vi "Periodic Tasks.vi"(8 "error in":errorcluster) -> ()   [LabVIEW 2013]
doc: "This VI runs in parallel to other tasks. It can contain as many user-defined periodic loops as you need. These can carry out PID or other sorts of timed response."
uses:
  <vilib>/Rock Robotics/SystemInterfaces/Utilities/FPGA_UtilitiesLED Source.ctl
  <vilib>/Rock Robotics/SystemInterfaces/Utilities/FPGA_UtilitiesLED State.ctl
  Robot Global Data.vi
  <vilib>/Rock Robotics/WPI/Joystick/WPI_JoystickGetSetRefNum.vi
  <vilib>/Utility/file.llb/Write To Spreadsheet File (DBL).vi
  <vilib>/Rock Robotics/WPI/DriverStation/WPI_DriverStationRobotMode2.ctl
  <vilib>/Rock Robotics/WPI/Camera/WPI_CameraWhite Balance Values.ctl
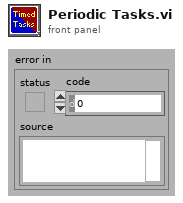
[diagram p1: front panel]
types:
  T1 = typedef "FPGA_UtilitiesLED State.ctl" = enum16{"Off", "On", "Toggle"}
  T2 = typedef "FPGA_UtilitiesLED Source.ctl" = enum16{"User LED", "FPGA LED"}
  T3 = typedef "WPI_DriverStationRobotMode2.ctl" = enum16{"Autonomous Disabled", "Autonomous Enabled", "Teleop Disabled", "Teleop Enabled", "Timeout", "Finish", "Test Disabled", "Test Enabled"}
  T4 = typedef "WPI_CameraWhite Balance Values.ctl" = enum16{"Auto", "Fixed indoor", "Fixed outdoor 1", "Fixed outdoor 2", "Fixed fluorescent 1", "Fixed fluorescent 2", "Hold current"}
  T5 = typedef "WPI_CameraDevRef.ctl" = cluster{"Camera Address":string, "CameraStatus":errorcluster, "Acquire Image Notifier":refnum<notifier>}
  T6 = typedef "WPI_JoystickDevRef.ctl" = cluster{"Device":T7}
  T7 = typedef "WPI_JoystickDeviceEnum.ctl" = enum16{"USB 1", "USB 2", "USB 3", "USB 4", "Kinect 1", "Kinect 2"}
  T8 = typedef "WPI_AnalogChannelDevRef.ctl" = cluster{"DevStatus":errorcluster, "Analog Module":T9, "Analog Channel":T10}
  T9 = typedef "FPGA_TypedefAnalogModule.ctl" = enum16{"Analog Module 1", "Analog Module 2"}
  T10 = typedef "FPGA_AIChannel.ctl" = enum8{"AI 1", "AI 2", "AI 3", "AI 4", "AI 5", "AI 6", "AI 7", "AI 8", "Invalid"}
  T11 = typedef "WPI_JoystickButtonState.ctl" = cluster{"Button 1":bool, "Button 2":bool, "Button 3":bool, "Button 4":bool, "Button 5":bool, "Button 6":bool, "Button 7":bool, "Button 8":bool, "Button 9":bool, "Button 10":bool, "Button 11":bool, "Button 12":bool}
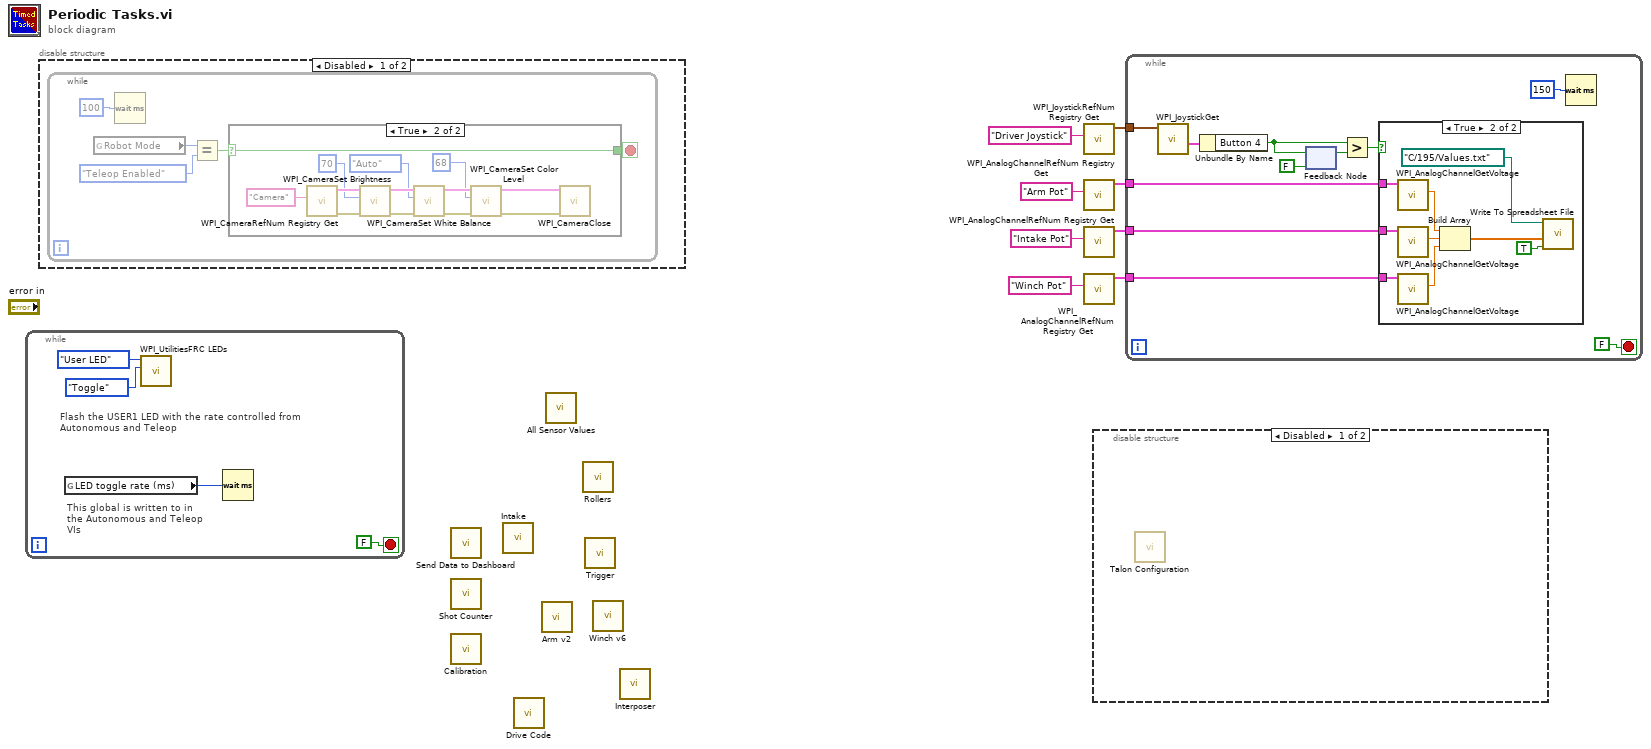
[diagram p0: block diagram]
diagram:
  n1 = while {
    stop <- FALSE stop-if-true
    # "This global is written to in the Autonomous and Teleop VIs"
    # "Flash the USER1 LED with the rate controlled from Autonomous and Teleop"
    n2 = global read "Robot Global Data.vi" "LED toggle rate (ms)"() -> (w9:u32)
    n3 = call <vilib>:"WPI_UtilitiesFRC LEDs.vi"("State"=FPGA_UtilitiesLED_State."Toggle", "LED Type"=FPGA_UtilitiesLED_Source."User LED") -> ()  [unwired: 1 in, 9 out]
    n4 = Wait (ms)(milliseconds to wait=w9) -> ()  [unwired: 1 out]
  }
  n5 = disable-structure shown="Disabled" {
    frame Disabled {
      n6 = while {
        stop <- w14 stop-if-true
        n7 = global read "Robot Global Data.vi" "Robot Mode"() -> (w16:T3)
        n8 = Wait (ms)(milliseconds to wait=u32 100) -> ()  [unwired: 1 out]
        n9 = Equal?(x=w16, y=WPI_DriverStationRobotMode2."Teleop Enabled") -> (x = y?=w17:bool)
        n10 = case shown="True" w17 {
          selector: w17 -> [w18 w31]
          tunnel: [w18 w31] -> w14
          frame False {
          }
          frame True {
            n11 = call <vilib>:"WPI_CameraRefNum Registry Get.vi"("refnum name"="Camera") -> ("error out"=w28:errorcluster, "CameraDevRef"=w29:T5)  [unwired: 9 in]
            n12 = call <vilib>:"WPI_CameraSet Brightness.vi"("error in (no error)"=w28, "Brightness"=70, "CameraDevRef"=w29) -> ("error out"=w24:errorcluster, "CameraDevRef Out"=w26:T5)  [unwired: 7 in]
            n13 = call <vilib>:"WPI_CameraSet White Balance.vi"("error in (no error)"=w24, "White Balance"=WPI_CameraWhite_Balance_Values."Auto", "CameraDevRef"=w26) -> ("error out"=w22:errorcluster, "CameraDevRef Out"=w23:T5)  [unwired: 7 in]
            n14 = call <vilib>:"WPI_CameraSet Color Level.vi"("error in (no error)"=w22, "Color Level"=68, "CameraDevRef"=w23) -> ("error out"=w20:errorcluster, "CameraDevRef Out"=w21:T5)  [unwired: 7 in]
            n15 = call <vilib>:"WPI_CameraClose.vi"("error in (no error)"=w20, "CameraDevRef"=w21) -> ()  [unwired: 9 in, 1 out]
          }
        }
      }
    }
    frame Enabled {
    }
  }
  n16 = call "Send Data to Dashboard.vi"() -> ()  [unwired: 12 in]
  n17 = call "Shot Counter.vi"() -> ()  [unwired: 12 in]
  n18 = call "Calibration.vi"() -> ()  [unwired: 12 in]
  n19 = call "Intake.vi"() -> ()  [unwired: 12 in]
  n20 = call "Drive Code.vi"() -> ()  [unwired: 12 in]
  n21 = call "Arm v2.vi"() -> ()  [unwired: 12 in]
  n22 = call "All Sensor Values.vi"() -> ()  [unwired: 12 in]
  n23 = call "Rollers.vi"() -> ()  [unwired: 12 in]
  n24 = call "Trigger.vi"() -> ()  [unwired: 12 in]
  n25 = call "Winch v6.vi"() -> ()  [unwired: 12 in]
  n26 = call "Interposer.vi"() -> ()  [unwired: 12 in]
  n27 = call <vilib>:"WPI_JoystickRefNum Registry Get.vi"("refnum name"="Driver Joystick") -> ("JoystickDevRef"=w8:T6)  [unwired: 9 in, 1 out]
  n28 = call <vilib>:"WPI_AnalogChannelRefNum Registry Get.vi"("refnum name"="Arm Pot") -> ("AIDeviceRef"=w7:T8)  [unwired: 9 in, 1 out]
  n29 = call <vilib>:"WPI_AnalogChannelRefNum Registry Get.vi"("refnum name"="Intake Pot") -> ("AIDeviceRef"=w4:T8)  [unwired: 9 in, 1 out]
  n30 = call <vilib>:"WPI_AnalogChannelRefNum Registry Get.vi"("refnum name"="Winch Pot") -> ("AIDeviceRef"=w3:T8)  [unwired: 9 in, 1 out]
  n31 = disable-structure shown="Disabled" {
    frame Disabled {
      n32 = call "Talon Configuration.vi"() -> ()  [unwired: 12 in]
    }
    frame Enabled {
    }
  }
  n33 = while {
    tunnel: w8 -> [w40]
    tunnel: w7 -> [w34]
    tunnel: w4 -> [w33]
    tunnel: w3 -> [w32]
    stop <- FALSE stop-if-true
    n34 = call <vilib>:"WPI_JoystickGet.vi"("JoystickDevRef"=w40) -> ("Buttons"=w39:T11)  [unwired: 4 in, 2 out]
    n35 = Unbundle By Name(w39) -> ("Button 4"=w37:bool)
    n36 = feedback-in #1(w37) -> ()
    n37 = feedback #1(FALSE ("Button 4")) -> (w38:bool)
    n38 = Greater?(x=w37, y=w38) -> (0:w35:bool)
    n39 = case shown="True" w35 {
      tunnel: w34 -> [_ w51]
      tunnel: w33 -> [_ w49]
      tunnel: w32 -> [_ w48]
      frame False {
      }
      frame True {
        n40 = call <vilib>:"WPI_AnalogChannelGetVoltage.vi"("AIDeviceRef"=w51) -> ("Voltage"=w50:dbl)  [unwired: 8 in, 2 out]
        n41 = call <vilib>:"WPI_AnalogChannelGetVoltage.vi"("AIDeviceRef"=w49) -> ("Voltage"=w47:dbl)  [unwired: 8 in, 2 out]
        n42 = call <vilib>:"WPI_AnalogChannelGetVoltage.vi"("AIDeviceRef"=w48) -> ("Voltage"=w46:dbl)  [unwired: 8 in, 2 out]
        n43 = Build Array(w50, w47, w46) -> (w44:dbl[])
        n44 = call-poly <vilib>:"Write To Spreadsheet File.vi"("append to file? (new file:F)"=TRUE, "1D data"=w44, "file path (dialog if empty)"=path "C:/195/Values.txt") -> ()  [unwired: 5 in, 1 out]
      }
    }
    n45 = Wait (ms)(milliseconds to wait=u32 150) -> ()  [unwired: 1 out]
  }
